vi "Multiplexer.vi"() -> ()   [LabVIEW 2018]
uses:
  <vilib>/Instr/_visa.llb/VISA Configure Serial Port (Instr).vi
panel:
  in  "Tab Control":enum32{"Manual", "Auto"}(tab)
  in  "Send Command":bool
  in  "Multiplexer Command":T1(ring)
  in  "Position":i32
  in  "Time between\nSwitches":u32=1000
  out "Last Sent Position":i32=1
  in  "Pattern":dbl[](array[numeric])=[0.0, 1.0]
  in  "stop":bool
  in  "Multiplexer\nPort":refnum<visa-resource-name>="COM10"
  out "Multiplexer Response":string="1"
  # "Minimum: 250"
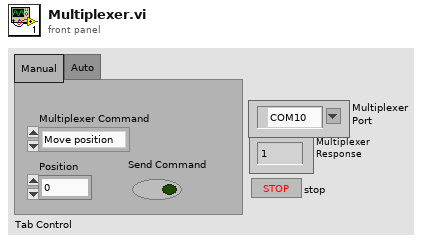
[diagram p1: front panel]
types:
  T1 = enum16{"Move position", "Get Status", "Get Program"}
  T2 = cluster{"baud rate":u32, "data bits":u16, "parity":enum16{"None", "Odd", "Even", "Mark", "Space"}, "stop bits":u16, "flow control":u16}
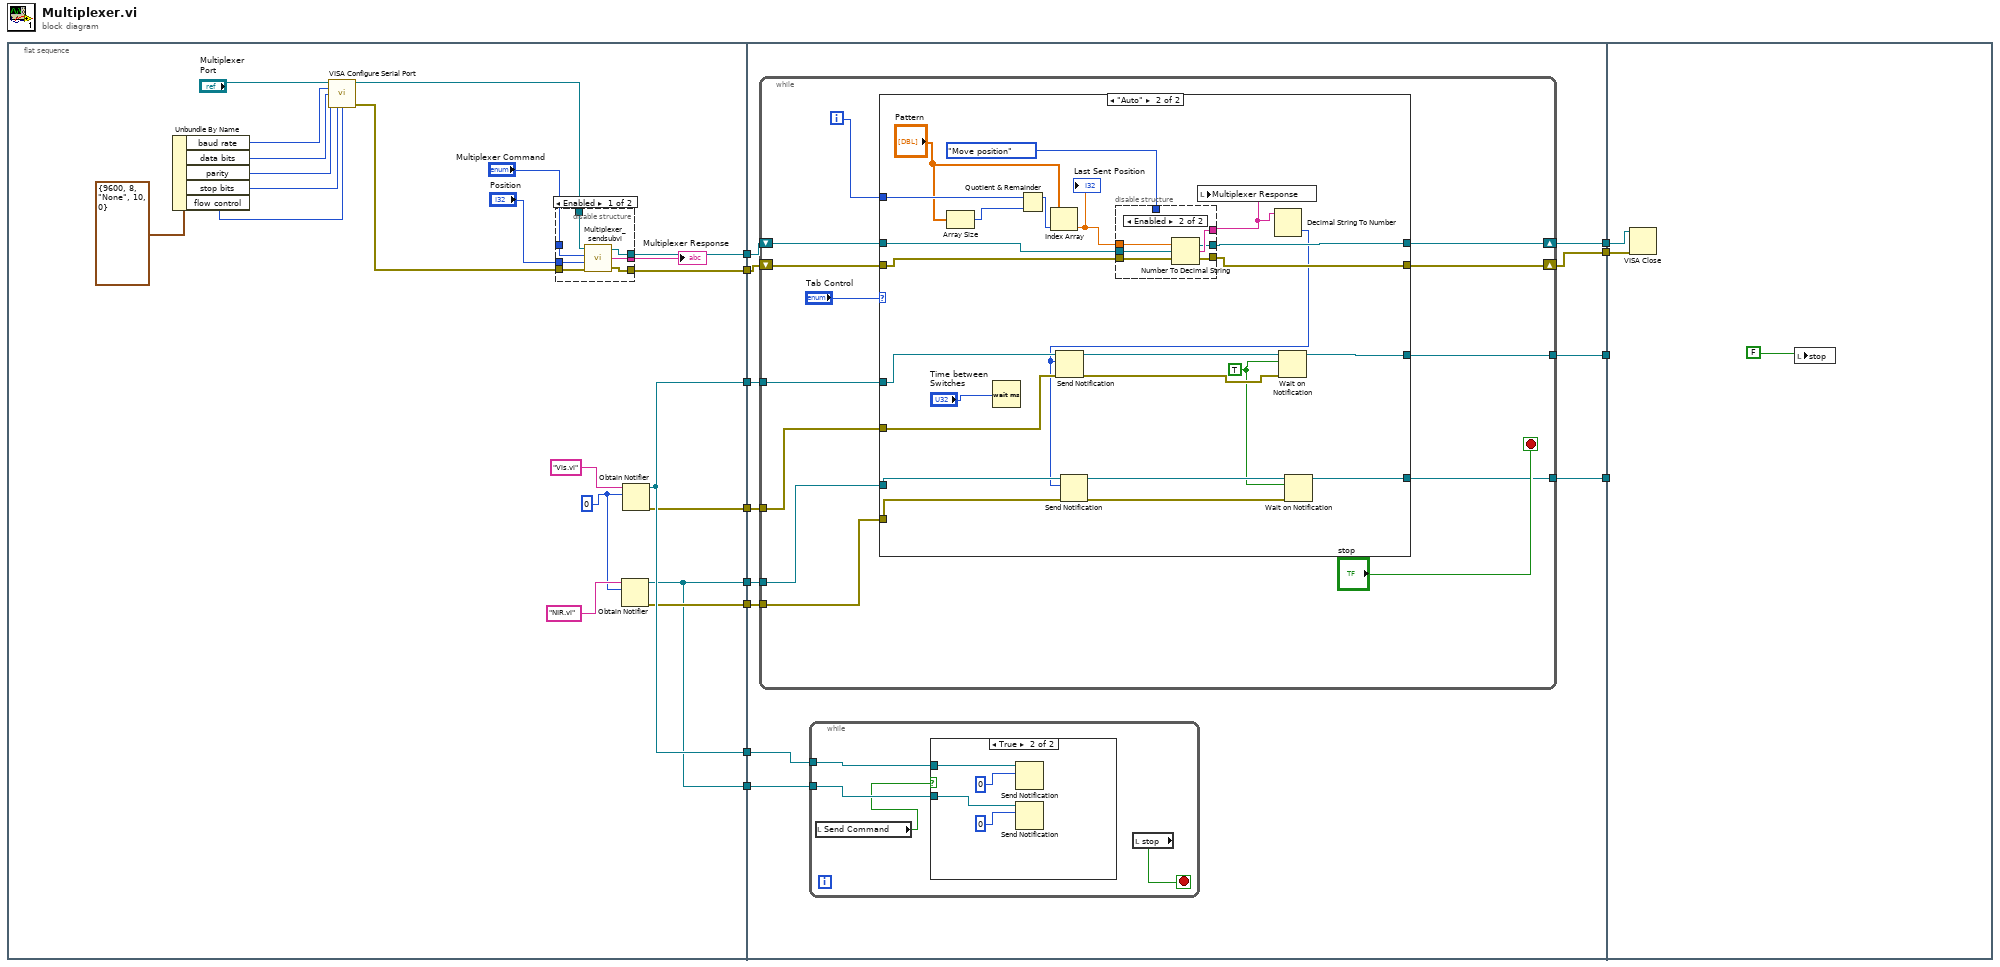
[diagram p0: block diagram]
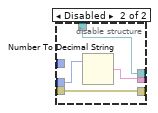
[diagram p2: hidden frame]
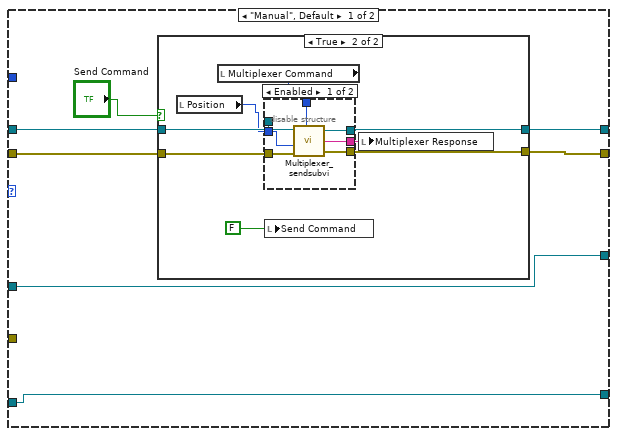
[diagram p4: hidden frame]
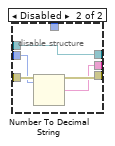
[diagram p6: hidden frame]
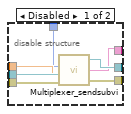
[diagram p7: hidden frame]
diagram:
  n1 = flat-sequence {
    tunnel: [w22] -> w12
    tunnel: [w21] -> w11
    tunnel: [w18] -> w8
    tunnel: [w18] -> w6
    tunnel: [w17] -> w5
    tunnel: [w13] -> w4
    tunnel: [w14] -> w3
    tunnel: [w13] -> w2
    tunnel: w12 -> [w56]
    tunnel: w11 -> [w55]
    tunnel: [w54] -> w10
    tunnel: [w53] -> w9
    tunnel: w8 -> [w52]
    tunnel: [w51] -> w7
    tunnel: w6 -> [w50]
    tunnel: w5 -> [w49]
    tunnel: w4 -> [w48]
    tunnel: w3 -> [w47]
    tunnel: w2 -> [w46]
    tunnel: [w45] -> w1
    tunnel: w10 -> [w142]
    tunnel: w9 -> [w141]
    tunnel: w7 -> [_]
    tunnel: w1 -> [_]
    frame #0 {
      w15 = 0 ("number")
      n2 = Unbundle By Name(T2 {"baud rate"=9600, "data bits"=8, "parity"=enum."None", "stop bits"=10, "flow control"=0} ("Serial Settings")) -> ("baud rate"=w31:u32, "data bits"=w30:u16, "parity"=w29:enum16{"None", "Odd", "Even", "Mark", "Space"}, "stop bits"=w28:u16, "flow control"=w27:u16)
      n3 = call-poly "VISA Configure Serial Port"("VISA resource name"="Multiplexer\nPort", "baud rate (9600)"=w31, "data bits (8)"=w30, "parity (0:none)"=w29, "stop bits (10: 1 bit)"=w28, "flow control (0:none)"=w27) -> ("VISA resource name out"=w20:refnum<visa-resource-name>, "error out"=w24:errorcluster)  [unwired: 3 in, 5 out]
      n4 = disable-structure shown="Enabled" {
        disable-tunnel: "Position" -> [w40 w44]
        disable-tunnel: "Multiplexer Command" -> [w39 _]
        disable-tunnel: w24 -> [w38 w42]
        disable-tunnel: w20 -> [w37 w41]
        disable-tunnel: [w36 w43] -> w23
        disable-tunnel: [w35 w41] -> w22
        disable-tunnel: [w34 w42] -> w21
        frame Enabled {
          n5 = call "Multiplexer_sendsubvi.vi"("error in (no error)"=w38, "Position"=w40, "Enum"=w39, "VISA resource name"=w37) -> ("error out"=w34:errorcluster, "Response"=w36:string, "VISA resource name out"=w35:refnum<visa-resource-name>)
        }
        frame Disabled {
          n6 = Number To Decimal String(number=w44) -> (decimal integer string=w43:string)  [unwired: 1 in]
        }
      }
      "Multiplexer Response" <- w23
      n7 = Obtain Notifier(name (unnamed)="NIR.vi", notification data type=w15) -> (notifier out=w13:refnum<notifier>, error out=w14:errorcluster)  [unwired: 2 in, 1 out]
      n8 = Obtain Notifier(name (unnamed)="Vis.vi", notification data type=w15) -> (notifier out=w18:refnum<notifier>, error out=w17:errorcluster)  [unwired: 2 in, 1 out]
    }
    frame #1 {
      n9 = while {
        shift-right: [w75] -> w54
        shift-left: w56 -> [w77]
        shift-right: [w74] -> w53
        shift-left: w55 -> [w76]
        tunnel: w52 -> [w71]
        tunnel: [w70] -> w51
        tunnel: w49 -> [w69]
        tunnel: w48 -> [w68]
        tunnel: w47 -> [w67]
        tunnel: [w66] -> w45
        i -> [w65]
        stop <- "stop" stop-if-true
        n10 = case shown="\"Auto\"" "Tab Control" {
          tunnel: w77 -> [w84 w129]
          tunnel: w76 -> [w83 w124]
          tunnel: [w82 w128] -> w75
          tunnel: [w81 w123] -> w74
          tunnel: w71 -> [w79 w121]
          tunnel: [w79 w122] -> w70
          tunnel: w69 -> [_ w118]
          tunnel: w68 -> [w78 w115]
          tunnel: w67 -> [_ w114]
          tunnel: [w78 w113] -> w66
          tunnel: w65 -> [_ w110]
          frame "Manual", Default {
            n11 = case shown="True" "Send Command" {
              tunnel: w84 -> [w86 w94]
              tunnel: w83 -> [w85 w93]
              tunnel: [w86 w92] -> w82
              tunnel: [w85 w91] -> w81
              frame False {
              }
              frame True {
                n12 = local read "Position"() -> (w87:i32)
                n13 = local read "Multiplexer Command"() -> (w90:T1)
                n14 = disable-structure shown="Enabled" {
                  disable-tunnel: w94 -> [w101 w104]
                  disable-tunnel: w93 -> [w100 w105]
                  disable-tunnel: [w99 w104] -> w92
                  disable-tunnel: [w98 w105] -> w91
                  disable-tunnel: w87 -> [w97 w102]
                  disable-tunnel: w90 -> [w96 _]
                  disable-tunnel: [w95 w103] -> w89
                  frame Enabled {
                    n15 = call "Multiplexer_sendsubvi.vi"("error in (no error)"=w100, "Position"=w97, "Enum"=w96, "VISA resource name"=w101) -> ("error out"=w98:errorcluster, "Response"=w95:string, "VISA resource name out"=w99:refnum<visa-resource-name>)
                  }
                  frame Disabled {
                    n16 = Number To Decimal String(number=w102) -> (decimal integer string=w103:string)  [unwired: 1 in]
                  }
                }
                n17 = local write "Send Command"(FALSE) -> ()
                n18 = local write "Multiplexer Response"(w89) -> ()
              }
            }
          }
          frame "Auto" {
            w112 = TRUE ("ignore previous (F)")
            n19 = Array Size(array="Pattern") -> (size(s)=w109:i32)
            n20 = Wait (ms)(milliseconds to wait="Time between\nSwitches") -> ()  [unwired: 1 out]
            n21 = Quotient & Remainder(x=w110, y=w109) -> (x-y*floor(x/y)=w108:i32)  [unwired: 1 out]
            n22 = Index Array(array="Pattern", index=w108) -> (element=w106:dbl)
            "Last Sent Position" <- w106
            n23 = disable-structure shown="Enabled" {
              disable-tunnel: w106 -> [w131 w140]
              disable-tunnel: T1."Move position" ("Multiplexer Command 2") -> [w130 _]
              disable-tunnel: w129 -> [w136 w137]
              disable-tunnel: w124 -> [w135 w139]
              disable-tunnel: [w134 w137] -> w128
              disable-tunnel: [w133 w139] -> w123
              disable-tunnel: [w132 w138] -> w125
              frame Disabled {
                n24 = call "Multiplexer_sendsubvi.vi"("error in (no error)"=w135, "Position"=w131, "Enum"=w130, "VISA resource name"=w136) -> ("error out"=w133:errorcluster, "Response"=w132:string, "VISA resource name out"=w134:refnum<visa-resource-name>)
              }
              frame Enabled {
                n25 = Number To Decimal String(number=w140) -> (decimal integer string=w138:string)  [unwired: 1 in]
              }
            }
            n26 = local write "Multiplexer Response"(w125) -> ()
            n27 = Decimal String To Number(string=w125) -> (number=w111:i32)  [unwired: 2 in, 1 out]
            n28 = Send Notification(notification=w111, notifier=w121, error in (no error)=w118) -> (notifier out=w120:refnum<notifier>, error out=w119:errorcluster)
            n29 = Send Notification(notification=w111, notifier=w115, error in (no error)=w114) -> (notifier out=w117:refnum<notifier>, error out=w116:errorcluster)
            n30 = Wait on Notification(notifier=w120, ignore previous (F)=w112, error in (no error)=w119) -> (notifier out=w122:refnum<notifier>)  [unwired: 1 in, 3 out]
            n31 = Wait on Notification(notifier=w117, ignore previous (F)=w112, error in (no error)=w116) -> (notifier out=w113:refnum<notifier>)  [unwired: 1 in, 3 out]
          }
        }
      }
      n32 = while {
        tunnel: w50 -> [w60]
        tunnel: w46 -> [w58]
        stop <- w59 stop-if-true
        n33 = local read "Send Command"() -> (w57:bool)
        n34 = case shown="True" w57 {
          tunnel: w60 -> [_ w64]
          tunnel: w58 -> [_ w61]
          frame False {
          }
          frame True {
            n35 = Send Notification(notification=0 ("number"), notifier=w64) -> ()  [unwired: 1 in, 2 out]
            n36 = Send Notification(notification=0 ("number"), notifier=w61) -> ()  [unwired: 1 in, 2 out]
          }
        }
        n37 = local read "stop"() -> (w59:bool)
      }
    }
    frame #2 {
      n38 = VISA Close(VISA resource name=w142, error in (no error)=w141) -> ()  [unwired: 1 out]
      n39 = local write "stop"(FALSE) -> ()
    }
  }
